vi "initAxis.vi"(0 "Error In":errorcluster caption="错误输入", 1 "handle":i32, 2 "ID":i32, 3 "modelName":string, 4 "AxisCount":i32) -> (5 "Error Out":errorcluster caption="错误输出", 6 "返回类型":i32)   [LabVIEW 2013, in "EM_CVx.lvlib"]
uses:
  EM_CVx.lvlib
  library/moverLibrary_x86.dll
  library/moverLibrary_x64.dll
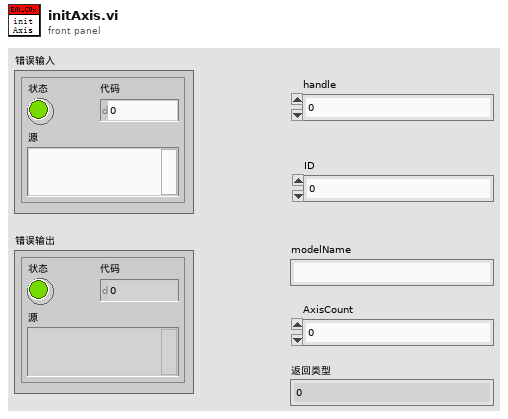
[diagram p1: front panel]
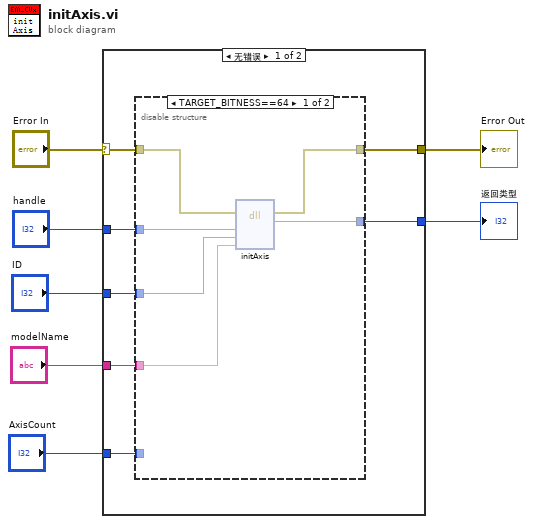
[diagram p0: block diagram]
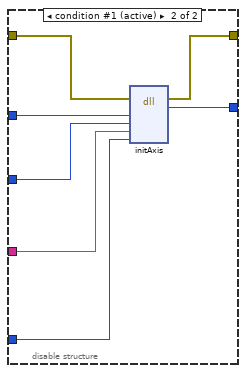
[diagram p2: hidden frame]
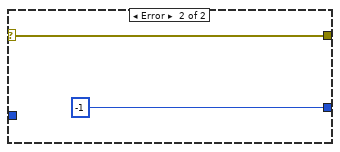
[diagram p3: hidden frame]
diagram:
  n1 = case shown="无错误" "Error In" {
    selector: "Error In" -> [w13 w29]
    tunnel: "modelName" -> [w14 _]
    tunnel: [w12 w29] -> w4
    tunnel: [w11 -1 ("返回类型")] -> w5
    tunnel: "ID" -> [w10 _]
    tunnel: "handle" -> [w9 _]
    tunnel: "AxisCount" -> [w8 _]
    frame No Error {
      n2 = disable-structure shown="TARGET_BITNESS==64" {
        disable-tunnel: w13 -> [w20 w27]
        disable-tunnel: w14 -> [w15 w26]
        disable-tunnel: [w19 w24] -> w12
        disable-tunnel: [w18 w25] -> w11
        disable-tunnel: w10 -> [w16 w23]
        disable-tunnel: w9 -> [w17 w22]
        disable-tunnel: w8 -> [_ w21]
        frame condition #0 {
          n3 = dll-call lib="E:/5-mover/4-labView/EM_CVx_2013/library/moverLibrary_x64.dll" fn="initAxis"(error in=w20, "handle"=w17, "ID"=w16, "serialName"=w15) -> (error out=w19:errorcluster, "return"=w18:i32)  [unwired: 5 in, 1 out]
        }
        frame condition #1 (active) {
          n4 = dll-call lib="E:/5-mover/4-labView/EM_CVx_2013/library/moverLibrary_x86.dll" fn="initAxis"(error in=w27, "handle"=w22, "ID"=w23, "serialName"=w26, "AxisCount"=w21) -> (error out=w24:errorcluster, "return"=w25:i32)  [unwired: 6 in, 1 out]
        }
      }
    }
    frame Error {
    }
  }
  "返回类型" <- w5
  "Error Out" <- w4
